vi "8HP_Process.vi"(0 "All samples in":sgl[][](array[numeric]), 1 "8HP Ch No":i16[](array[numeric]), 2 "Analysis info Index":i32[](array[numeric]), 3 "Sampling Rate":dbl, 4 "Probe Number":i32) -> ()   [LabVIEW 2020]
uses:
  <vilib>/Analysis/NI_AALBase.lvlib
  <vilib>/Analysis/baseanly.llb/Mean (DBL).vi
  Sub_vis/Upload Data.ctl
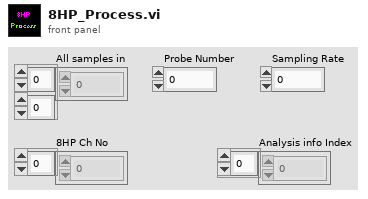
[diagram p1: front panel]
types:
  T1 = typedef "Upload Data.ctl" = enum16{"Voltage Array", "Time Trace Cluster"}
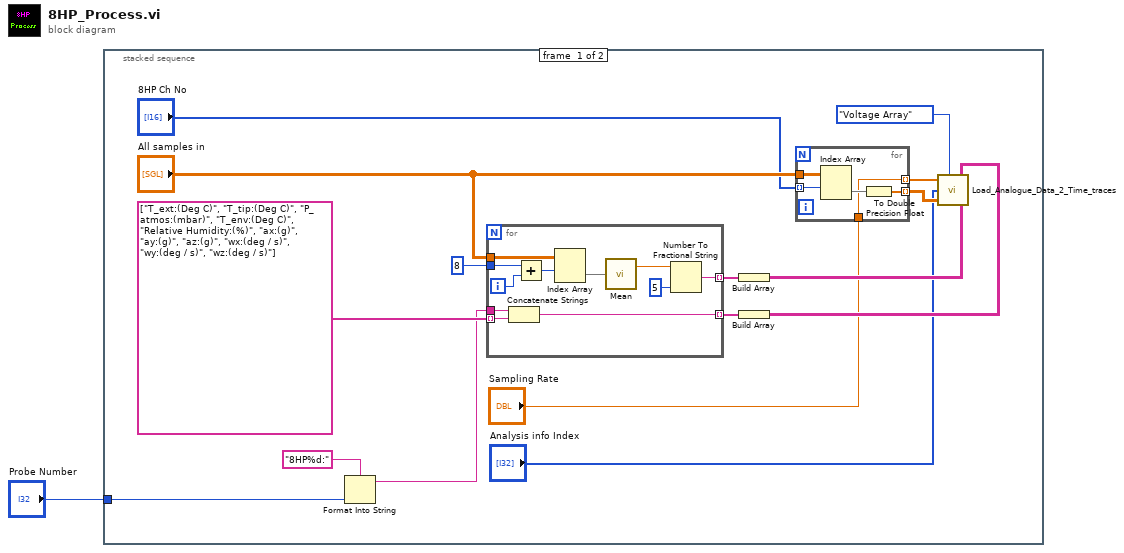
[diagram p0: block diagram]
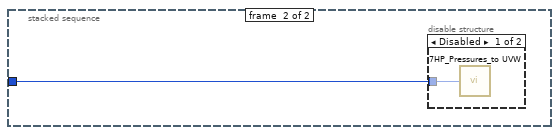
[diagram p2: hidden frame]
diagram:
  n1 = stacked-sequence {
    tunnel: "Probe Number" -> [w4 w34]
    frame #0 {
      n2 = Format Into String(format string="8HP%d:", w4) -> (resulting string=w5:string)  [unwired: 2 in, 1 out]
      n3 = for {
        tunnel: "All samples in" -> [w28]
        tunnel: 8 -> [w26]
        tunnel: w5 -> [w24]
        tunnel: string[] ["T_ext:(Deg C)", "T_tip:(Deg C)", "P_atmos:(mbar)", "T_env:(Deg C)", "Relative Humidity:(%)", "ax:(g)", "ay:(g)", "az:(g)", "wx:(deg / s)", "wy:(deg / s)", "wz:(deg / s)"] -> [w23] mode=indexing
        tunnel: [w19] -> w14 mode=indexing
        tunnel: [w18] -> w13 mode=indexing
        i -> [w27]
        n4 = Concatenate Strings(w24, w23) -> (w18:string)
        n5 = Add(x=w26, y=w27) -> (x+y=w25:i32)
        n6 = Index Array(array=w28, index (row)=w25) -> (element=w22:sgl[])  [unwired: 1 in]
        n7 = call-poly <vilib>:"Mean.vi"("X"=w22) -> ("mean"=w21:dbl)  [unwired: 1 out]
        n8 = Number To Fractional String(number=w21, precision (6)=i16 5) -> (F-format string=w19:string)  [unwired: 2 in]
      }
      n9 = Build Array(w14) -> (w16:string[][])
      n10 = Build Array(w13) -> (w15:string[][])
      n11 = for {
        tunnel: "8HP Ch No" -> [w32] mode=indexing
        tunnel: "All samples in" -> [w33]
        tunnel: "Sampling Rate" -> [w29]
        tunnel: [w30] -> w9 mode=indexing
        tunnel: [w29] -> w10 mode=indexing
        n12 = Index Array(array=w33, index (row)=w32) -> (element=w31:sgl[])  [unwired: 1 in]
        n13 = To Double Precision Float(number=w31) -> (double precision float=w30:dbl[])
      }
      n14 = call "Load_Analogue_Data_2_Time_traces.vi"("Sampling Rate (Hz)"=w10, "Mode"=Upload_Data."Voltage Array", "Index"="Analysis info Index", "Voltage Array"=w9, "Metadata Names"=w15, "Metadata Values"=w16) -> ()  [unwired: 1 in]
    }
    frame #1 {
      n15 = disable-structure shown="Disabled" {
        disable-tunnel: w34 -> [w35 _]
        frame Disabled {
          n16 = call "7HP_Pressures_to UVW.vi"("Probe Number"=w35) -> ()
        }
        frame Enabled {
        }
      }
    }
  }
